vi "Configure Math Function Display Mode.vi"(8 "error in (no error)":errorcluster, 9 "Math Display Mode (0: Normal)":i32(ring) items=["Normal", "Average", "Max Hold", "Min Hold"], 10 "Math Function Index (1: Math Function 1)":i32(ring)=1 items=["Math Function 1"=1, "Math Function 2"=2, "Math Function 3"=3, "Math Function 4"=4], 11 "VISA resource name":refnum<visa-resource-name>) -> (0 "error out":errorcluster, 3 "VISA resource name out":refnum<visa-resource-name>)   [LabVIEW 2015, in "Agilent 2000 3000 X-Series.lvlib"]
doc: "Selects one of the math function display modes.\n\nNotes:\nThis command is part of the FUNCtion subsystem that controls the math functions in the oscilloscope.\nThe 3000 T Series has a dedicated FFT function. The FFT subsystem controls the FFT function in the oscilloscope. For FFT Display use the <b>Configure FFT Display</b> VI."
uses:
  <instrlib>/Agilent 2000 3000 X-Series/Agilent 2000 3000 X-Series.lvlib
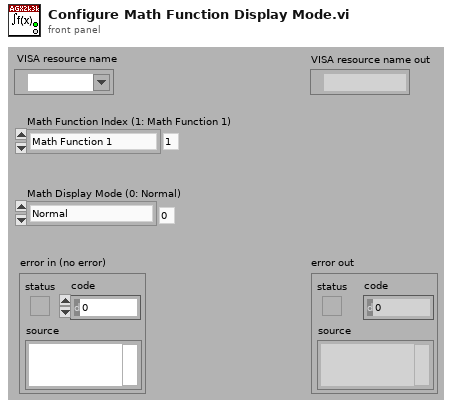
[diagram p1: front panel]
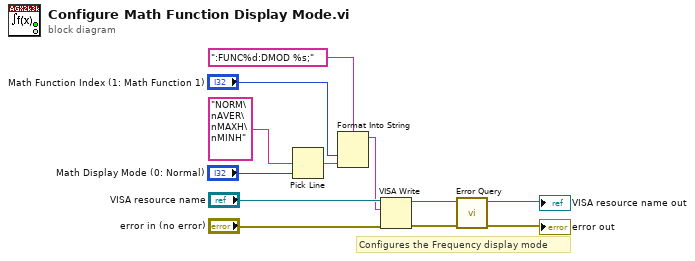
[diagram p0: block diagram]
diagram:
  # "Configures the Frequency display mode"
  n1 = Pick Line(multi-line string="NORM\nAVER\nMAXH\nMINH", line index="Math Display Mode (0: Normal)") -> (output string=w1:string)  [unwired: 1 in]
  n2 = Format Into String(format string=":FUNC%d:DMOD %s;" ("multi-line string"), "Math Function Index (1: Math Function 1)", w1) -> (resulting string=w2:string)  [unwired: 2 in, 1 out]
  n3 = VISA Write(VISA resource name="VISA resource name", write buffer=w2, error in (no error)="error in (no error)") -> (VISA resource name out=w12:refnum<visa-resource-name>, error out=w11:errorcluster)  [unwired: 1 out]
  n4 = call <instrlib>:"Error Query.vi"("error in (no error)"=w11, "VISA resource name"=w12) -> ("error out"=→"error out":errorcluster, "VISA resource name out"=→"VISA resource name out":refnum<visa-resource-name>)  [unwired: 8 out]
